vi "SENS_CORR_COLL_SESS_CONN_PORT_SEL.vi"(0 "VISA IN":refnum<visa-resource-name>, 2 "ConnType":string(combo), 5 "error in":errorcluster, 7 "Channel":i32=1, 9 "Session":i32, 11 "Port":i32) -> (14 "VISA Out":refnum<visa-resource-name>, 19 "error out":errorcluster)   [LabVIEW 2018, in "PNA-X.lvlib"]
doc: "SENSe:CORRection:COLLect:GUIDed:STEPs?\n(Read-only) Returns the number of measurement steps required to complete the current guided calibration. This command is sent after the SENS:CORR:COLL:GUID:INIT, SENS:CORR:COLL:GUID:CONN:PORT and SENS:CORR:COLL:GUID:CKIT:PORT commands.\n \nExamples\n SENS:CORR:COLL:GUID:STEP?\nsense2:correction:collect:guided:steps?\n \nReturn Type\n Numeric\n \nDefault\n Not Applicable"
uses:
  PNA-X.lvlib
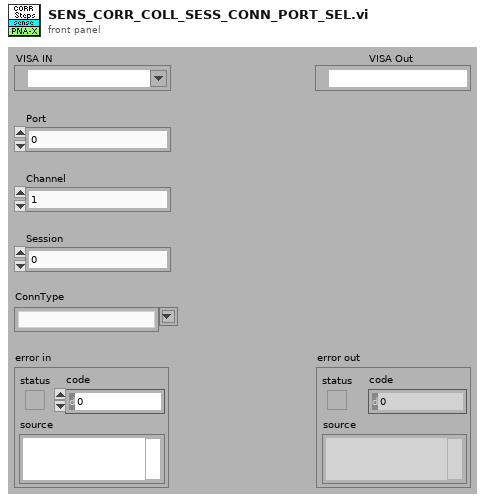
[diagram p1: front panel]
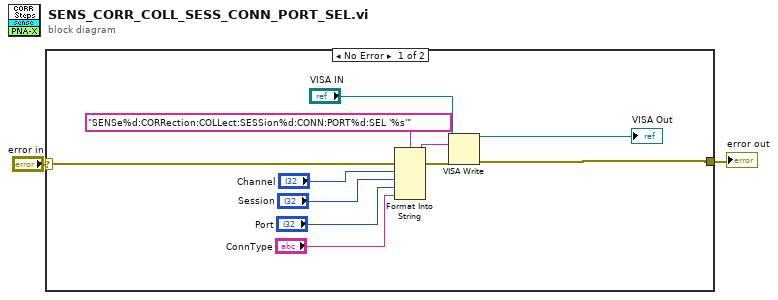
[diagram p0: block diagram]
diagram:
  n1 = case shown="No Error" "error in" {
    selector: "error in" -> [w13 w14]
    tunnel: [w7 w14] -> w1
    frame No Error {
      n2 = Format Into String(format string="SENSe%d:CORRection:COLLect:SESSion%d:CONN:PORT%d:SEL '%s'" ("Cmdline"), error in=w13, "Channel", "Session", "Port", "ConnType") -> (resulting string=w11:string, error out=w12:errorcluster)  [unwired: 1 in]
      n3 = VISA Write(VISA resource name="VISA IN", write buffer=w11, error in (no error)=w12) -> (VISA resource name out=→"VISA Out":refnum<visa-resource-name>, error out=w7:errorcluster)  [unwired: 1 out]
    }
    frame Error {
    }
  }
  "error out" <- w1
